vi "test simple.vi"(8 "error in (no error)":errorcluster, 11 "MyTestCase in":refnum<class "MyTestCase.lvclass">) -> (0 "error out":errorcluster, 3 "MyTestCase out":refnum<class "MyTestCase.lvclass">)   [LabVIEW 2020, in "MyTestCase.lvclass"]
uses:
  MyTestCase.lvclass
  C:/Program Files/National Instruments/LabVIEW 2020/vi.lib/addons/_JKI Toolkits/VI Tester/TestCase.llb/TestCase.lvclass
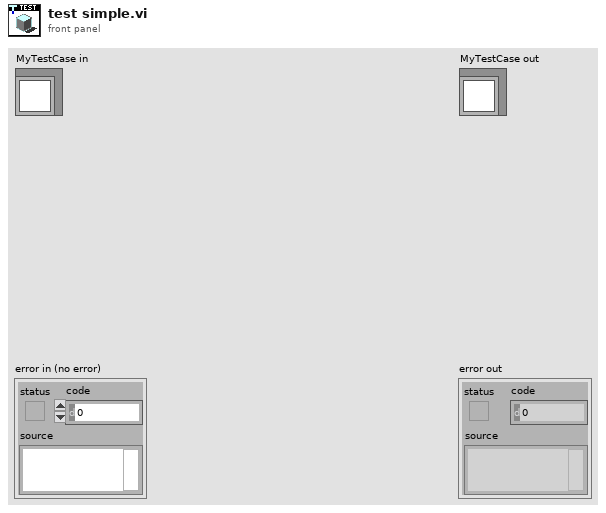
[diagram p1: front panel]
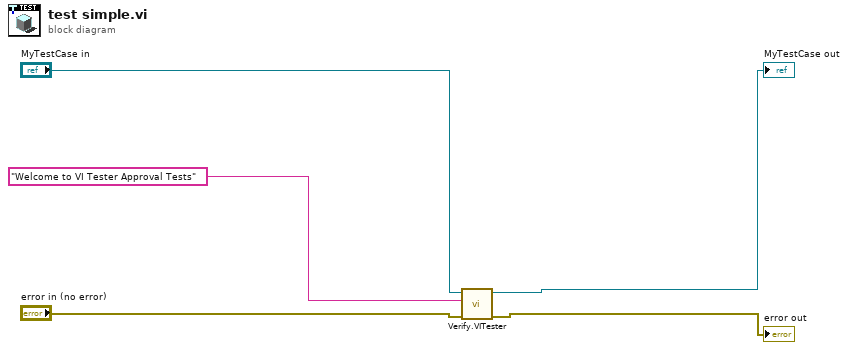
[diagram p0: block diagram]
diagram:
  n1 = call "Verify.VITester.vi"("error in (no error)"="error in (no error)", "Test Data"="Welcome to VI Tester Approval Tests", "TestCase in"="MyTestCase in") -> ("error out"=→"error out":errorcluster, "TestCase out"=→"MyTestCase out":refnum<class "MyTestCase.lvclass">)  [unwired: 7 in]
